vi "Stage.vi"() -> ()   [LabVIEW 2019]
panel:
  out "Stage":dbl
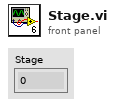
[diagram p1: front panel]
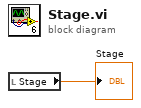
[diagram p0: block diagram]
diagram:
  n1 = local read "Stage"() -> (→"Stage":dbl)
